vi "Find Instances.vi"(0 "MVA Comms VI in":refnum<class "MVA Comms VI Instance.lvclass">, 11 "error in (no error)":errorcluster) -> (4 "MVA Comms VI out":refnum<class "MVA Comms VI Instance.lvclass">, 6 "Instances":refnum<class "MVA Comms VI Instance.lvclass">[](array[class]), 15 "error out":errorcluster)   [LabVIEW 2020, in "MVA Message Mapper.lvlib" / "MVA Comms VI Instance.lvclass"]
uses:
  <vilib>/gpm_packages/@cs/Bus-message-mapper/Source/support/MVA Comms/MVA Comms VI Instance.lvclass
  <vilib>/Utility/traverseref.llb/TRef TravTarget.ctl
  <vilib>/gpm_packages/@cs/Bus-message-mapper/Source/support/MVA Comms/MVA Comms VI Instance.lvclass/MVA Comms VI Instance.ctl
  <vilib>/gpm_packages/@cs/Bus-message-mapper/Source/support/MVA Comms/Accessors/Write MVA Coms VI Instance.vi
  <vilib>/gpm_packages/@cs/Bus-message-mapper/Source/support/MVA Comms/Accessors/Read Project Reference.vi
  <vilib>/gpm_packages/@cs/Bus-message-mapper/Source/support/MVA Comms/Accessors/Read MVA Coms VI Name.vi
  <vilib>/Utility/traverseref.llb/VI Scripting - Traverse.lvlib
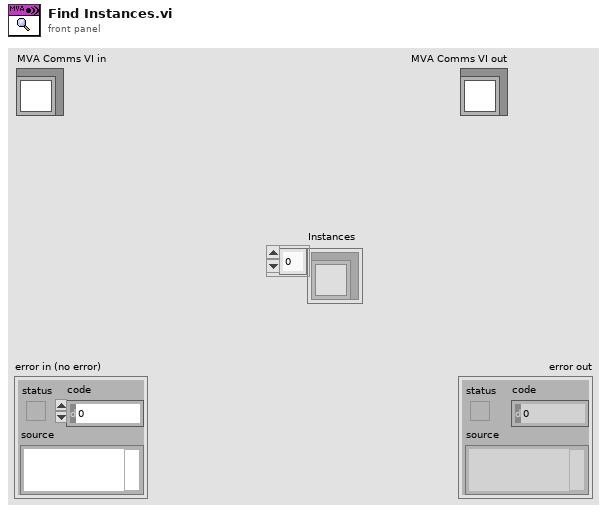
[diagram p1: front panel]
types:
  T1 = typedef "TRef TravTarget.ctl" = enum16{"FP", "BD", "Other"}
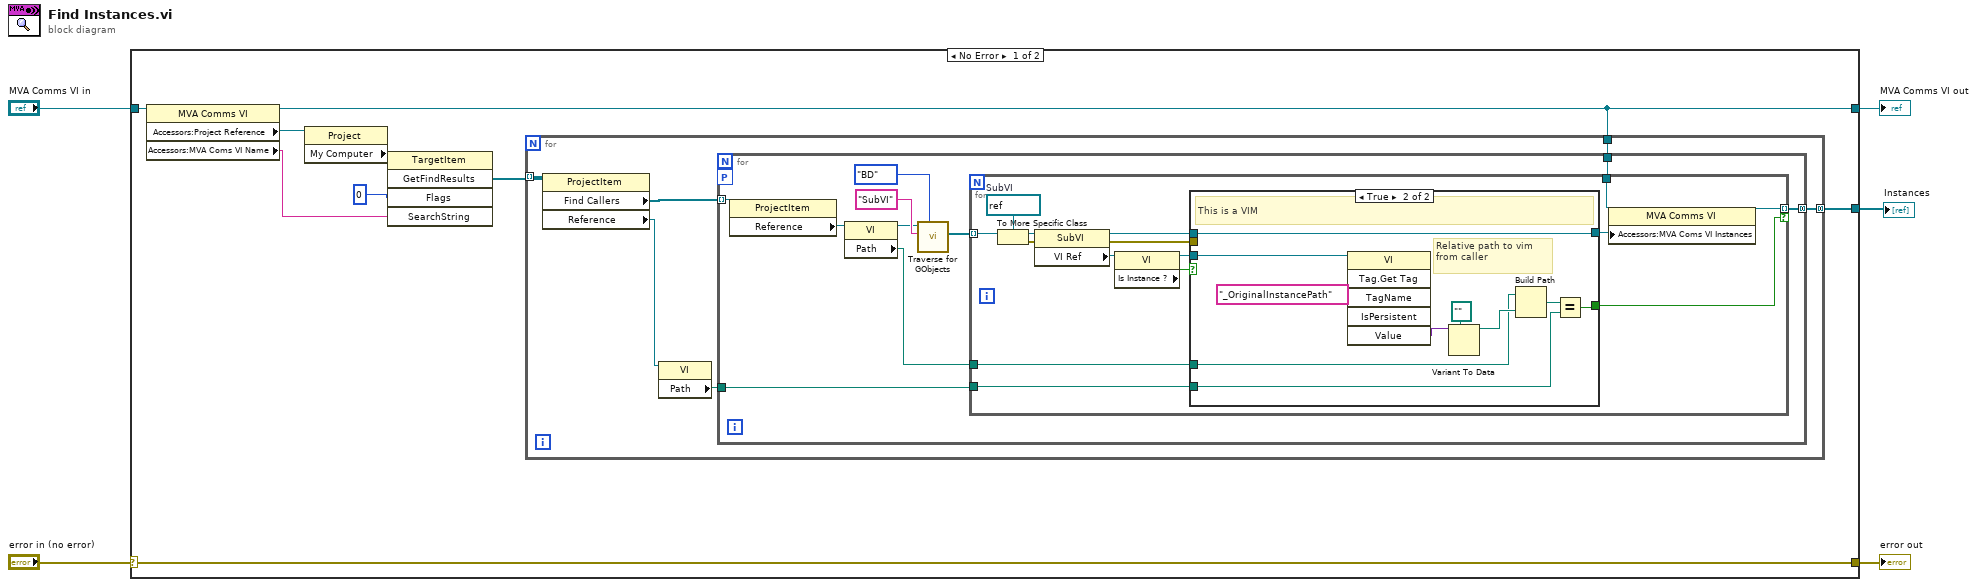
[diagram p0: block diagram]
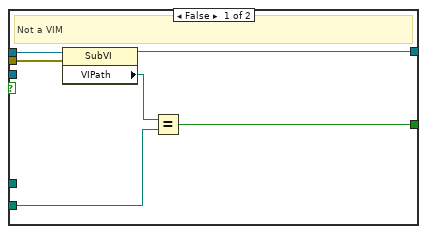
[diagram p2: hidden frame]
diagram:
  n1 = case shown="No Error" "error in (no error)" {
    selector: "error in (no error)" -> [w14 w62]
    tunnel: [w14 w62] -> w4
    tunnel: [w9 w61] -> w2
    tunnel: "MVA Comms VI in" -> [w10 w61]
    tunnel: [w6 _] -> w1
    frame No Error {
      n2 = property class="MVA Comms VI"(reference=w10) -> (reference out=w9:refnum<class "MVA Comms VI Instance.lvclass">, "Accessors:Project Reference"=w8:refnum<vi>, "Accessors:MVA Coms VI Name"=w7:string)  [unwired: 1 in, 1 out]
      n3 = property class="Project"(reference=w8) -> ("My Computer"=w11:refnum<vi>)  [unwired: 1 in, 2 out]
      n4 = invoke class="TargetItem" method="GetFindResults"(reference=w11, "Flags"=0, "SearchString"=w7) -> ("GetFindResults"=w13:refnum<vi>[])  [unwired: 2 in, 4 out]
      n5 = for {
        tunnel: w13 -> [w18] mode=indexing
        tunnel: [w20] -> w6 mode=concatenating
        tunnel: w9 -> [w16]
        n6 = property class="ProjectItem"(reference=w18) -> ("Find Callers"=w19:refnum<vi>[], "Reference"=w15:refnum<vi>)  [unwired: 1 in, 2 out]
        n7 = property class="VI"(reference=w15) -> ("Path"=w17:path)  [unwired: 1 in, 2 out]
        n8 = for {
          tunnel: w19 -> [w26] mode=indexing
          tunnel: [w27] -> w20 mode=concatenating
          tunnel: w17 -> [w25]
          tunnel: w16 -> [w24]
          workers-P: _ -> [_]
          n9 = property class="ProjectItem"(reference=w26) -> ("Reference"=w23:refnum<vi>)  [unwired: 1 in, 2 out]
          n10 = property class="VI"(reference=w23) -> (reference out=w22:refnum<vi>, "Path"=w21:path)  [unwired: 1 in, 1 out]
          n11 = call <vilib>:"Traverse for GObjects.vi"("Traverse Target"=TRef_TravTarget."BD", "Class Name"="SubVI", "VI Refnum"=w22) -> ("References"=w28:refnum<vi>[])  [unwired: 5 in, 3 out]
          n12 = for {
            tunnel: w28 -> [w42] mode=indexing
            tunnel: [w37] -> w27 mode=indexing if=w41
            tunnel: w25 -> [w40]
            tunnel: w24 -> [w39]
            tunnel: w21 -> [w31]
            w43 = refnum<vi> refnum  # SubVI
            n13 = To More Specific Class(target class=w43, reference=w42) -> (specific class reference=w36:refnum<vi>, error out=w44:errorcluster)  [unwired: 1 in]
            n14 = property class="SubVI"(reference=w36) -> (reference out=w34:refnum<vi>, "VI Ref"=w35:refnum<vi>)  [unwired: 1 in, 1 out]
            n15 = property class="VI"(reference=w35) -> (reference out=w32:refnum<vi>, "Is Instance ?"=w33:bool)  [unwired: 1 in, 1 out]
            n16 = case shown="True" w33 {
              tunnel: w34 -> [w50 w60]
              tunnel: w44 -> [w49 _]
              tunnel: [w47 w52] -> w41
              tunnel: w40 -> [w46 w51]
              tunnel: [w45 w60] -> w38
              tunnel: w32 -> [_ w59]
              tunnel: w31 -> [_ w54]
              frame False {
                # "Not a VIM"
                n17 = property class="SubVI"(reference=w50, error in=w49) -> (reference out=w45:refnum<vi>, "VIPath"=w48:path)  [unwired: 1 out]
                n18 = Equal?(x=w48, y=w46) -> (x = y?=w47:bool)
              }
              frame True {
                # "Relative path to vim\nfrom caller"
                # "This is a VIM"
                n19 = invoke class="VI" method="Tag.Get Tag"(reference=w59, "TagName"="_OriginalInstancePath" ("Tag Name")) -> ("Value"=w57:variant)  [unwired: 4 in, 5 out]
                n20 = Variant To Data(type=path "", Variant=w57) -> (data=w55:path)  [unwired: 1 in, 1 out]
                n21 = Build Path(base path=w54, name or relative path=w55) -> (appended path=w53:path)
                n22 = Equal?(x=w53, y=w51) -> (x = y?=w52:bool)
              }
            }
            n23 = property class="MVA Comms VI"(reference=w39, "Accessors:MVA Coms VI Instances"=w38) -> (reference out=w37:refnum<class "MVA Comms VI Instance.lvclass">)  [unwired: 1 in, 1 out]
          }
        }
      }
    }
    frame Error {
    }
  }
  "error out" <- w4
  "MVA Comms VI out" <- w2
  "Instances" <- w1
